vi "Reset Supply.vi"(8 "error in":errorcluster, 11 "6700C in":refnum<class "6700C.lvclass">) -> (0 "error out":errorcluster, 3 "6700C out":refnum<class "6700C.lvclass">)   [LabVIEW 2019, in "6700C.lvlib" / "6700C.lvclass"]
uses:
  Library/6700C.lvclass
  Library/6700C.lvclass/6700C.ctl
  builds/Instruments/PowerSupply.lvlibp/Library/PowerSupply.lvclass
  <instrlib>/Agilent N6700 Series/Agilent N6700 Series.lvlib
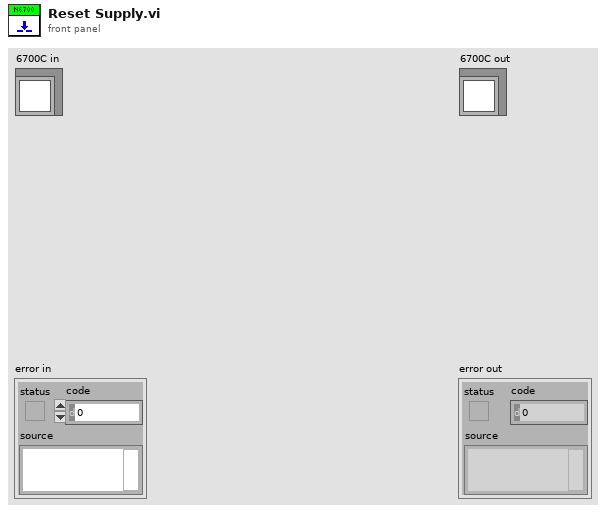
[diagram p1: front panel]
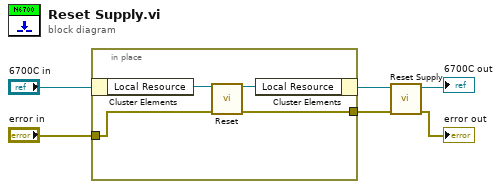
[diagram p0: block diagram]
diagram:
  n1 = in-place {
    in-place-border: "error in" -> [w7]
    in-place-border: [w8] -> w3
    n2 = in-place-cluster #1("6700C in") -> ("Local Resource"=w10:refnum<visa-resource-name>)
    n3 = call <instrlib>:"Reset.vi"("VISA resource name"=w10, "error in (no error)"=w7) -> ("VISA resource name out"=w9:refnum<visa-resource-name>, "error out"=w8:errorcluster)  [unwired: 12 in]
    n4 = in-place-cluster #1("Local Resource"=w9) -> (w4:refnum<class "6700C.lvclass">)
  }
  n5 = call-parent "Reset Supply.vi"("error in"=w3, "PowerSupply in"=w4) -> ("error out"=→"error out":errorcluster, "PowerSupply out"=→"6700C out":refnum<class "6700C.lvclass">)  [unwired: 8 in]
